vi "RemoteControlForFTJH.vi"() -> ()   [LabVIEW 2020]
uses:
  LMH-PS4/Private/Type Defs/Indicators/Controller.ctl
  LMH-PS4/Private/Type Defs/Indicators/Square.ctl
  LMH-PS4/Private/Type Defs/Indicators/X.ctl
  LMH-PS4/Private/Type Defs/Indicators/Circle.ctl
  LMH-PS4/Private/Type Defs/Indicators/Triangle.ctl
  LMH-PS4/Private/Type Defs/Indicators/L1.ctl
  LMH-PS4/Private/Type Defs/Indicators/R1.ctl
  LMH-PS4/Private/Type Defs/Indicators/Share.ctl
  LMH-PS4/Private/Type Defs/Indicators/Options.ctl
  LMH-PS4/Private/Type Defs/Indicators/PS.ctl
  LMH-PS4/Private/Type Defs/Indicators/Pad_Button.ctl
  LMH-PS4/Private/Type Defs/Indicators/Dpad.ctl
  LMH-PS4/Private/Type Defs/Indicators/Slider.ctl
  <vilib>/Platform/TimedLoop/XDataNode/timing_clust.ctl
  <vilib>/Platform/TimedLoop/XDataNode/nitl_modes.ctl
  <vilib>/Platform/TimedLoop/XDataNode/wakeup.ctl
  <vilib>/CISH Robotics/L4VMX TitanQuad/Motor ID.ctl
  <vilib>/CISH Robotics/L4VMX VMXpi/Type Def/VMX Channel Index.ctl
  servoName.ctl
  <vilib>/CISH Robotics/L4VMX VMXpi/Digital Output/Digital Output.lvclass
  <vilib>/CISH Robotics/L4VMX TitanQuad/TitanQuad.lvclass
  <vilib>/CISH Robotics/L4VMX VMXpi/PWM Generator/PWM Generator.lvclass
  <vilib>/platform/TimedLoop/XDataNode/XDataNode.xnode
  <vilib>/ReMiSYS Technology/RemoteToolkit/Receiver/Receiver.lvclass
  LMH-PS4/LMH-PS4.lvlib
  <vilib>/CISH Robotics/L4VMX VMXpi/Power/Power.lvclass
  <vilib>/Platform/TimedLoop/XDataNode/XDNodeRunTimeDep.lvlib
  <vilib>/CISH Robotics/L4VMX VMXpi/L4VMX.lvlib
  <vilib>/CISH Robotics/L4VMX VMXpi/Utilities/Utilities.lvclass
  <vilib>/CISH Robotics/L4VMX VMXpi/Digital Input/Digital Input.lvclass
panel:
  in  "NormalizeTo":dbl=450.0
  out "Start":bool
  out "Voltage":sgl
  out "Error Out":errorcluster
  in  "Stop":bool
  out "Received?":bool
  out "PS4 Controller":T1={"Square Button"=FALSE, "X Button"=FALSE, "Circle Button"=FALSE, "Triangle Button"=FALSE, "L1"=FALSE, "R1"=FALSE, "Share Button"=FALSE, "Options Button"=FALSE, "PS Button"=FALSE, "Pad Button"=FALSE, "D-Pad"=5, "L2"=0, "R2"=0, "Thumbstick_Left"={[], []}, "Thumbstick_Right"={[], []}} {"R2" scale=-32768.0..32767.0; "L2" scale=-32768.0..32767.0}
  # "ss"
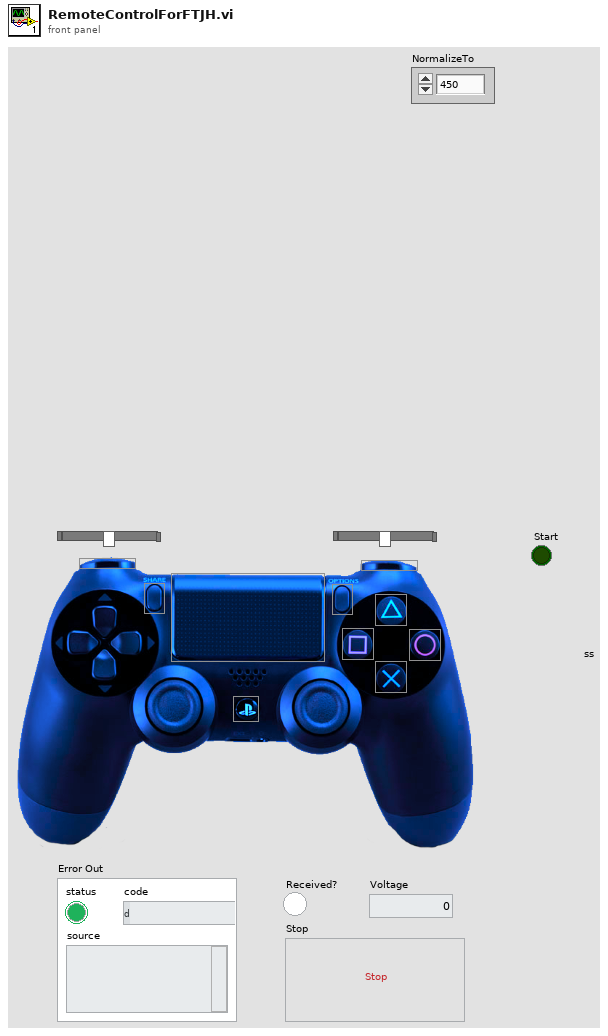
[diagram p1: front panel]
types:
  T1 = typedef "LMH-PS4.lvlib/Controller.ctl" = cluster{"Square Button":T2, "X Button":T3, "Circle Button":T4, "Triangle Button":T5, "L1":T6, "R1":T7, "Share Button":T8, "Options Button":T9, "PS Button":T10, "Pad Button":T11, "D-Pad":T12, "L2":T13, "R2":T13, "Thumbstick_Left":cluster{i32[], i32[]}, "Thumbstick_Right":cluster{i32[], i32[]}}
  T2 = typedef "LMH-PS4.lvlib/Square.ctl" = bool
  T3 = typedef "LMH-PS4.lvlib/X.ctl" = bool
  T4 = typedef "LMH-PS4.lvlib/Circle.ctl" = bool
  T5 = typedef "LMH-PS4.lvlib/Triangle.ctl" = bool
  T6 = typedef "LMH-PS4.lvlib/L1.ctl" = bool
  T7 = typedef "LMH-PS4.lvlib/R1.ctl" = bool
  T8 = typedef "LMH-PS4.lvlib/Share.ctl" = bool
  T9 = typedef "LMH-PS4.lvlib/Options.ctl" = bool
  T10 = typedef "LMH-PS4.lvlib/PS.ctl" = bool
  T11 = typedef "LMH-PS4.lvlib/Pad_Button.ctl" = bool
  T12 = typedef "LMH-PS4.lvlib/Dpad.ctl" = u16
  T13 = typedef "LMH-PS4.lvlib/Slider.ctl" = i32
  T14 = typedef "L4VMX.lvlib/VMX Channel Index.ctl" = enum16{"0", "1", "2", "3", "4", "5", "6", "7", "8", "9", "10", "11", "12", "13", "14", "15", "16", "17", "18", "19", "20", "21", "22", "23", "24", "25", "26", "27", "28", "29", "30", "31", "32", "33"}
  T15 = typedef "TitanQuad.lvlib/TitanQuad.lvclass/Motor ID.ctl" = enum16{"M0", "M1", "M2", "M3"}
  T16 = typedef "XDNodeRunTimeDep.lvlib/timing_clust.ctl" = cluster{"Expected End [f-1]":u64, "Actual End [f-1]":u64, "Finished Late? [f-1]":bool, "Expected End [i-1]":u64, "Actual End [i-1]":u64, "Finished Late? [i-1]":bool, "Expected Start [i]":u64, "Actual Start [i]":u64, "Expected Start [f]":u64, "Actual Start [f]":u64, "Source Name":string, "Structure Name":string, "Period":i64, "Deadline":i64, "Offset":i64, "Start":i64, "Priority":i32, "Timeout":i32, "Mode":T17, "Wakeup Reason":T18, "Error":errorcluster, "Source Type":string, "Secondary Source Type":string, "Global End Time":u64, "Global Start Time":u64, "Frame Duration":u64, "Iteration Duration":u64, "Assigned CPU":i32, "I/O Scan Engine Mode":u32}
  T17 = typedef "XDNodeRunTimeDep.lvlib/nitl_modes.ctl" = enum32{"No Change", "Process missed periods, maintain original phase", "Discard missed periods, maintain original phase", "Process missed periods, ignore original phase", "Discard missed periods, ignore original phase"}
  T18 = typedef "XDNodeRunTimeDep.lvlib/wakeup.ctl" = enum32{"Normal", "Aborted", "Asynchronous wakeup", "Timing source error", "Timed loop error", "Timeout"}
  T19 = typedef "servoName.ctl" = enum16{"Servo1", "Servo2", "Servo3", "Servo4"}
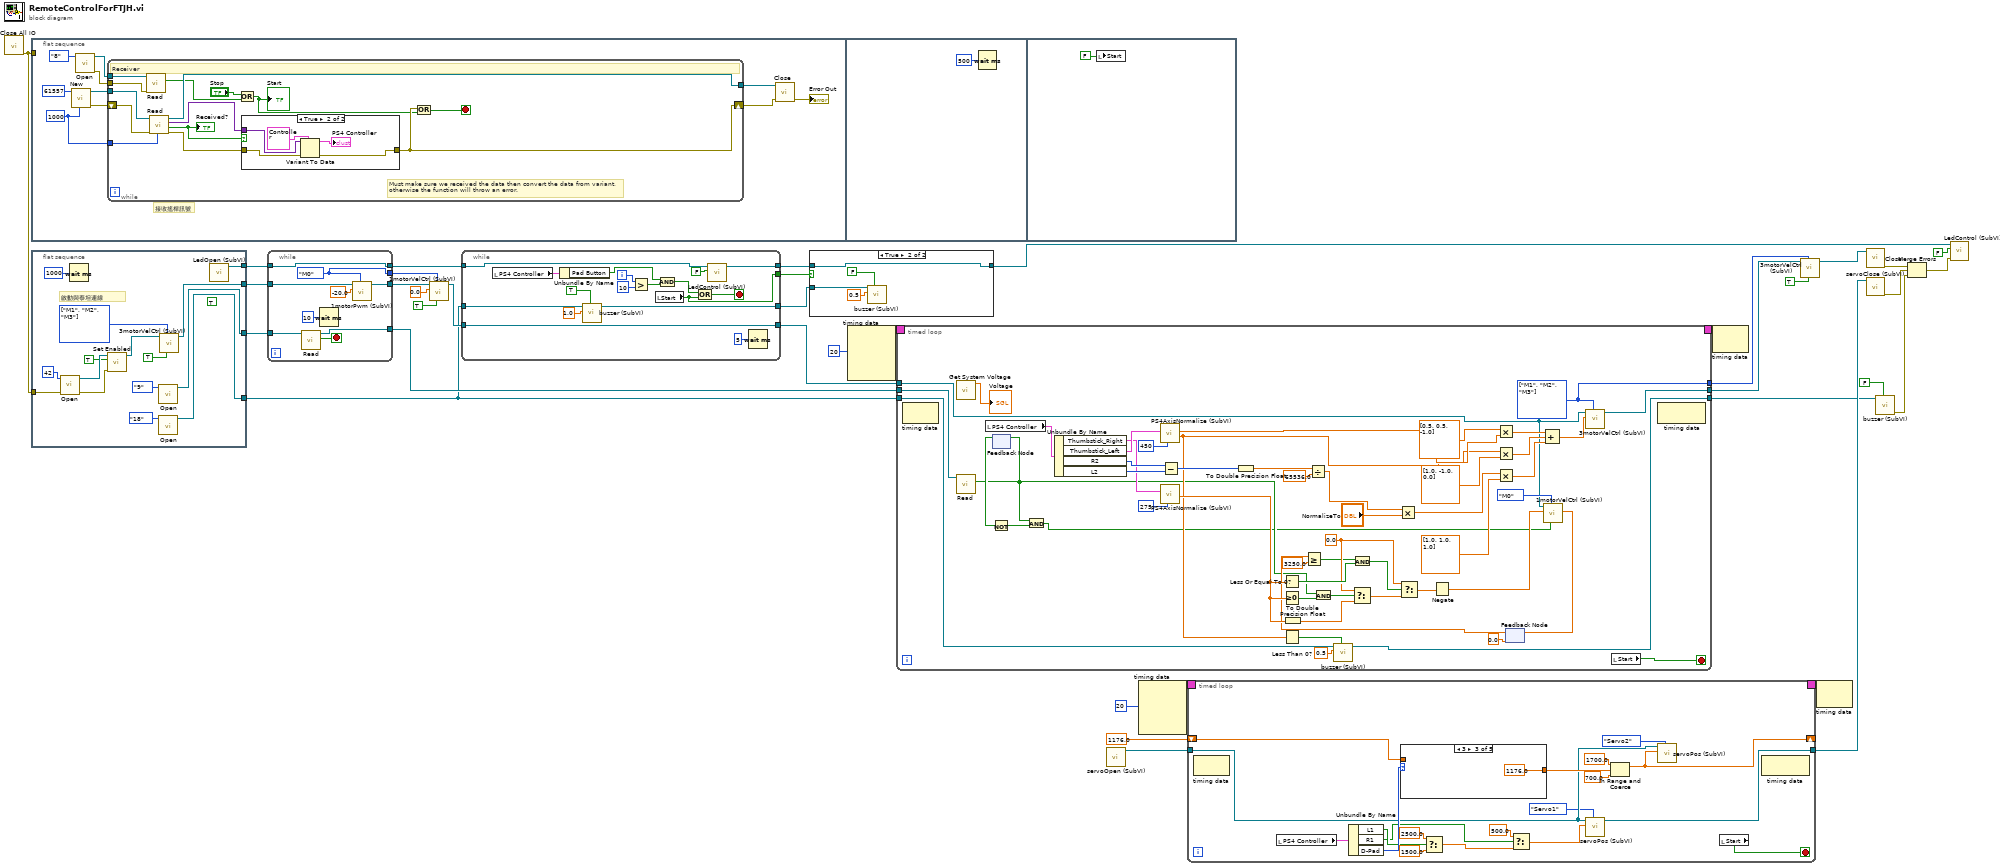
[diagram p0: block diagram]
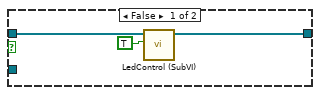
[diagram p2: hidden frame]
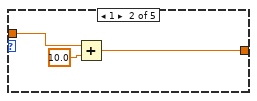
[diagram p4: hidden frame]
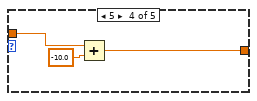
[diagram p5: hidden frame]
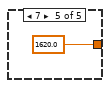
[diagram p6: hidden frame]
diagram:
  n1 = call <vilib>:"Close All IO.vi"() -> ("Error Out"=w1:errorcluster)  [unwired: 11 in]
  n2 = flat-sequence {
    tunnel: w1 -> [_]
    frame #0 {
      w43 = 1000 ("Timeout ms (25000)")
      # "接收搖桿訊號"
      n3 = call <vilib>:"New.vi"("Timeout ms (25000)"=w43, "Port (61557)"=u16 61557) -> ("Error Out"=w47:errorcluster, "Receiver Ref."=w46:refnum<class "Receiver.lvclass">)  [unwired: 8 in]
      n4 = call <vilib>:"Open.vi"("VMX Channel Index"=VMX_Channel_Index."8") -> ("Error Out"=w38:errorcluster, "Digital Input Object"=w39:refnum<class "Digital Input.lvclass">)  [unwired: 9 in]
      n5 = while {
        shift-right: [w54] -> w45
        shift-left: w47 -> [w61]
        tunnel: w46 -> [w60]
        tunnel: [w59] -> w44
        tunnel: w43 -> [w58]
        tunnel: w39 -> [w52]
        tunnel: w38 -> [w51]
        stop <- w57 stop-if-true
        # "Must make sure we received the data then convert the data from variant,\notherwise the function will throw an error."
        # "Receiver"
        n6 = call <vilib>:"Read.vi"("Error In"=w51, "Digital Input Object"=w52) -> ("Value"=w50:bool)  [unwired: 7 in, 2 out]
        n7 = call <vilib>:"Read.vi"("Timeout ms (1000)"=w58, "Error In"=w61, "Receiver Ref."=w60) -> ("Error Out"=w56:errorcluster, "Received?"=w53:bool, "Value"=w55:variant, "Receiver Ref."=w59:refnum<class "Receiver.lvclass">)  [unwired: 5 in]
        "Received?" <- w53
        n8 = Or(x="Stop", y=w50) -> (x .or. y?=w48:bool)
        "Start" <- w48
        n9 = case shown="True" w53 {
          tunnel: w56 -> [w62 w67]
          tunnel: w55 -> [_ w66]
          tunnel: [w62 w65] -> w54
          frame False {
          }
          frame True {
            n10 = Variant To Data(error in=w67, type=T1 {"Square Button"=FALSE, "X Button"=FALSE, "Circle Button"=FALSE, "Triangle Button"=FALSE, "L1"=FALSE, "R1"=FALSE, "Share Button"=FALSE, "Options Button"=FALSE, "PS Button"=FALSE, "Pad Button"=FALSE, "D-Pad"=0, "L2"=-32768, "R2"=-32768, "Thumbstick_Left"={[0, 0], [0, 0]}, "Thumbstick_Right"={[0, 0], [0, 0]}} ("PS4 Controller"), Variant=w66) -> (data=→"PS4 Controller":T1, error out=w65:errorcluster)
          }
        }
        n11 = Or(x=w54, y=w48) -> (x .or. y?=w57:bool)
      }
      n12 = call <vilib>:"Close.vi"("Error In"=w45, "Receiver Ref."=w44) -> ("Error Out"=→"Error Out":errorcluster)  [unwired: 9 in]
    }
    frame #1 {
      n13 = Wait (ms)(milliseconds to wait=u32 500) -> ()  [unwired: 1 out]
    }
    frame #2 {
      n14 = local write "Start"(FALSE ("Stop")) -> ()
    }
  }
  n15 = flat-sequence {
    tunnel: w1 -> [w79]
    tunnel: [w77] -> w10
    tunnel: [w75] -> w12
    tunnel: [w72] -> w3
    tunnel: [w70] -> w2
    frame #0 {
      (unwired) TRUE ("reset Encoder")
      w76 = T15[] [enum."M1", enum."M2", enum."M3"] items=["M0", "M1", "M2", "M3"] ("motorPort [M0, M1, M2]")
      # "啟動與泰坦連線"
      n16 = call <vilib>:"Open.vi"("Error In"=w79, "Titan ID (42)"=u8 42) -> ("Error Out"=w83:errorcluster, "TitanQuad Object"=w84:refnum<class "TitanQuad.lvclass">)  [unwired: 8 in]
      n17 = Wait (ms)(milliseconds to wait=u32 1000) -> ()  [unwired: 1 out]
      n18 = call <vilib>:"Set Enabled.vi"("Error In"=w83, "Enable"=TRUE, "TitanQuad Object"=w84) -> ("TitanQuad Object"=w74:refnum<class "TitanQuad.lvclass">)  [unwired: 7 in, 1 out]
      n19 = call <vilib>:"Open.vi"("VMX Channel Index"=VMX_Channel_Index."9") -> ("Digital Input Object"=w72:refnum<class "Digital Input.lvclass">)  [unwired: 9 in, 1 out]
      n20 = call <vilib>:"Open.vi"("VMX Channel Index"=VMX_Channel_Index."18") -> ("Digital Output Object"=w70:refnum<class "Digital Output.lvclass">)  [unwired: 9 in, 1 out]
      n21 = call "3motorVelCtrl (SubVI).vi"("reset Encoder"=TRUE, "motorPort [M0, M1, M2]"=w76, "TitanQuad in"=w74) -> ("TitanQuad out"=w77:refnum<class "TitanQuad.lvclass">)  [unwired: 6 in, 2 out]
      n22 = call "LedOpen (SubVI).vi"() -> ("LedRef"=w75:refnum<class "Digital Output.lvclass">[])  [unwired: 10 in, 1 out]
    }
  }
  n23 = while {
    tunnel: [w93] -> w13
    tunnel: w12 -> [w93]
    tunnel: [w90] -> w8
    tunnel: w10 -> [w92]
    tunnel: [w89] -> w9
    tunnel: w3 -> [w88]
    tunnel: [w87] -> w4
    stop <- w86 stop-if-true
    w89 = Motor_ID."M0" ("Motor ID")
    n24 = call <vilib>:"Read.vi"("Digital Input Object"=w88) -> ("Value"=w86:bool, "Digital Input Object"=w87:refnum<class "Digital Input.lvclass">)  [unwired: 8 in, 1 out]
    n25 = Wait (ms)(milliseconds to wait=u32 10) -> ()  [unwired: 1 out]
    n26 = call "1motorPwm (SubVI).vi"("Motor ID"=w89, "motorPwmSpeed"=-20.0, "TitanQuad in"=w92) -> ("TitanQuad out"=w90:refnum<class "TitanQuad.lvclass">)  [unwired: 6 in, 2 out]
  }
  n27 = call "1motorVelCtrl (SubVI).vi"("reset Encoder"=TRUE, "Motor ID"=w9, "motorSpeed (deg/s)"=0.0, "TitanQuad in"=w8) -> ("TitanQuad out"=w7:refnum<class "TitanQuad.lvclass">)  [unwired: 3 in, 4 out]
  n28 = while {
    tunnel: [w102] -> w30
    tunnel: w13 -> [w101]
    tunnel: [w99] -> w23
    tunnel: w2 -> [w98]
    tunnel: [w96] -> w14
    tunnel: [w94] -> w11
    tunnel: w7 -> [w94]
    i -> [w107]
    stop <- w103 stop-if-true
    n29 = local read "PS4 Controller"() -> (w110:T1)
    n30 = Unbundle By Name(w110) -> ("Pad Button"=w108:T11)
    n31 = call "buzzer (SubVI).vi"("BuzzerOn"=TRUE, "Time Target (s)"=1.0, "Digital Output in"=w98) -> ("Digital Output out"=w96:refnum<class "Digital Output.lvclass">)  [unwired: 7 in, 1 out]
    n32 = Greater?(x=w107, y=10) -> (0:w105:bool)
    n33 = local read "Start"() -> (w102:bool)
    n34 = And(x=w108, y=w105) -> (x .and. y?=w104:T11)
    n35 = Or(x=w104, y=w102) -> (x .or. y?=w103:T11)
    n36 = call "LedControl (SubVI).vi"("Red/Green [T/F]"=FALSE, "LedRef"=w101) -> ("LedRef"=w99:refnum<class "Digital Output.lvclass">[])  [unwired: 8 in, 1 out]
    n37 = Wait (ms)(milliseconds to wait=u32 5) -> ()  [unwired: 1 out]
  }
  n38 = case shown="True" w30 {
    tunnel: w23 -> [w112 w117]
    tunnel: [w111 w117] -> w20
    tunnel: w14 -> [_ w115]
    frame False {
      n39 = call "LedControl (SubVI).vi"("Red/Green [T/F]"=TRUE, "LedRef"=w112) -> ("LedRef"=w111:refnum<class "Digital Output.lvclass">[])  [unwired: 8 in, 1 out]
    }
    frame True {
      n40 = call "buzzer (SubVI).vi"("BuzzerOn"=FALSE, "Time Target (s)"=0.5, "Digital Output in"=w115) -> ()  [unwired: 7 in, 2 out]
    }
  }
  n41 = node-c288(i64 20 ("Period")) -> (w37:T16)  [unwired: 3 in]
  n42 = timed-loop {
    timing: w37 -> [_]
    timing-out: [_] -> w36
    tunnel: w4 -> [w158]
    tunnel: [w148] -> w29
    tunnel: [w147] -> w26
    tunnel: w2 -> [w130]
    tunnel: [w127] -> w17
    tunnel: w11 -> [w125]
    stop <- w169 stop-if-true
    w147 = T15[] [enum."M1", enum."M2", enum."M3"] items=["M0", "M1", "M2", "M3"] ("motorPort [M0, M1, M2]")
    w152 = 0.0 ("t")
    n43 = node-c288() -> ()  [unwired: 1 in, 1 out]
    n44 = call <vilib>:"Get System Voltage.vi"() -> ("Voltage"=→"Voltage":sgl)  [unwired: 10 in, 1 out]
    n45 = call <vilib>:"Read.vi"("Digital Input Object"=w158) -> ("Value"=w122:bool)  [unwired: 8 in, 2 out]
    n46 = local read "PS4 Controller"() -> (w167:T1)
    n47 = feedback-in #1(w122) -> ()
    n48 = feedback #1() -> (w123:bool)  [unwired: 1 in]
    n49 = Not(x=w123) -> (.not. x?=w124:bool)
    n50 = And(x=w122, y=w124) -> (x .and. y?=w121:bool)
    n51 = Unbundle By Name(w167) -> ("Thumbstick_Right"=w140:cluster{i32[], i32[]}, "Thumbstick_Left"=w143:cluster{i32[], i32[]}, "R2"=w166:T13, "L2"=w165:T13)
    n52 = call "PS4AxisNormalize (SubVI).vi"("NormalizeTo"=450, "PS4 Thumbstick"=w143) -> ("Y"=w129:dbl, "X"=w142:dbl)  [unwired: 8 in]
    n53 = call "PS4AxisNormalize (SubVI).vi"("NormalizeTo"=275, "PS4 Thumbstick"=w140) -> ("Y"=w138:dbl)  [unwired: 8 in, 1 out]
    n54 = Subtract(x=w166, y=w165) -> (x-y=w131:T13)
    n55 = To Double Precision Float(number=w131) -> (double precision float=w133:dbl)
    n56 = Less Or Equal To 0?(x=w138) -> (x <= 0?=w154:bool)
    n57 = Greater Or Equal To 0?(x=w138) -> (x >= 0?=w157:bool)
    n58 = Less Than 0?(x=w129) -> (x < 0?=w128:bool)
    n59 = To Double Precision Float(number=w138) -> (double precision float=w137:dbl)
    n60 = Divide(x=w133, y=65536.0) -> (x/y=w120:dbl)
    n61 = And(x=w122, y=w157) -> (x .and. y?=w156:bool)
    n62 = call "buzzer (SubVI).vi"("BuzzerOn"=w128, "Time Target (s)"=0.5, "Digital Output in"=w130) -> ("Digital Output out"=w127:refnum<class "Digital Output.lvclass">)  [unwired: 7 in, 1 out]
    n63 = Select(t=w152, s=w156, f=w137) -> (s? t:f=w155:dbl)
    n64 = Multiply(x=w120, y="NormalizeTo") -> (x*y=w118:dbl)
    n65 = Multiply(x=dbl[] [0.5, 0.5, -1.0], y=w142) -> (x*y=w161:dbl[])
    n66 = Multiply(x=w129, y=dbl[] [1.0, -1.0, 0.0]) -> (x*y=w160:dbl[])
    n67 = Multiply(x=w118, y=dbl[] [1.0, 1.0, 1.0]) -> (x*y=w164:dbl[])
    n68 = feedback #2(0.0 ("Enc (deg)")) -> (w135:dbl)
    n69 = Greater Or Equal?(x=w135, y=3250.0) -> (x >= y?=w150:bool)
    n70 = And(x=w150, y=w154) -> (x .and. y?=w153:bool)
    n71 = Select(t=w152, s=w153, f=w155) -> (s? t:f=w145:dbl)
    n72 = Negate(x=w145) -> (-x=w144:dbl)
    n73 = call "1motorVelCtrl (SubVI).vi"("reset Encoder"=w121, "Motor ID"=Motor_ID."M0", "motorSpeed (deg/s)"=w144, "TitanQuad in"=w125) -> ("Enc (deg)"=w136:dbl)  [unwired: 3 in, 4 out]
    n74 = feedback-in #2(w136) -> ()
    n75 = Compound Arithmetic op=ADD(w161, w160, w164) -> (w149:dbl[])
    n76 = call "3motorVelCtrl (SubVI).vi"("motorPort [M0, M1, M2]"=w147, "motorSpeed [M0, M1, M2] (deg/s)"=w149, "TitanQuad in"=w125) -> ("TitanQuad out"=w148:refnum<class "TitanQuad.lvclass">)  [unwired: 6 in, 2 out]
    n77 = local read "Start"() -> (w169:bool)
    n78 = node-c288() -> ()  [unwired: 1 in, 1 out]
  }
  n79 = call "servoOpen (SubVI).vi"() -> ("ServosRef"=w25:refnum<class "PWM Generator.lvclass">[])  [unwired: 10 in, 1 out]
  n80 = node-c288(i64 20 ("Period")) -> (w34:T16)  [unwired: 3 in]
  n81 = timed-loop {
    timing: w34 -> [_]
    timing-out: [_] -> w33
    shift-right: [w172] -> _
    shift-left: 1176.0 ("y") -> [w187]
    tunnel: w25 -> [w178]
    tunnel: [w177] -> w24
    stop <- w190 stop-if-true
    n82 = node-c288() -> ()  [unwired: 1 in, 1 out]
    n83 = local read "PS4 Controller"() -> (w189:T1)
    n84 = Unbundle By Name(w189) -> ("L1"=w183:T6, "R1"=w175:T7, "D-Pad"=w188:T12)
    n85 = case shown="3" w188 {
      tunnel: w187 -> [w191 w194 _ w198 _]
      tunnel: [w191 w192 1176.0 ("y") w196 1620.0 ("y")] -> w185
      frame 0, Default {
      }
      frame 1 {
        n86 = Add(x=w194, y=10.0) -> (x+y=w192:dbl)
      }
      frame 3 {
      }
      frame 5 {
        n87 = Add(x=w198, y=-10.0) -> (x+y=w196:dbl)
      }
      frame 7 {
      }
    }
    n88 = Select(t=2500.0, s=w183, f=1500.0 ("lower limit")) -> (s? t:f=w181:dbl)
    n89 = Select(t=500.0, s=w175, f=w181) -> (s? t:f=w174:dbl)
    n90 = call "servoPos (SubVI).vi"("Servos"=servoName."Servo1", "ServoPosition (us)"=w174, "ServosRef in"=w178) -> ("ServosRef out"=w177:refnum<class "PWM Generator.lvclass">[])  [unwired: 7 in, 1 out]
    n91 = In Range and Coerce(upper limit=1700.0, x=w185, lower limit=700.0) -> (coerced(x)=w172:dbl)  [unwired: 1 out]
    n92 = call "servoPos (SubVI).vi"("Servos"=servoName."Servo2", "ServoPosition (us)"=w172, "ServosRef in"=w178) -> ()  [unwired: 7 in, 2 out]
    n93 = local read "Start"() -> (w190:bool)
    n94 = node-c288() -> ()  [unwired: 1 in, 1 out]
  }
  n95 = node-c288(w36) -> ()  [unwired: 1 out]
  n96 = call "3motorVelCtrl (SubVI).vi"("reset Encoder"=TRUE, "motorPort [M0, M1, M2]"=w26, "TitanQuad in"=w29) -> ("TitanQuad out"=w28:refnum<class "TitanQuad.lvclass">)  [unwired: 6 in, 2 out]
  n97 = node-c288(w33) -> ()  [unwired: 1 out]
  n98 = call <vilib>:"Close.vi"("TitanQuad Object"=w28) -> ("Error Out"=w22:errorcluster)  [unwired: 10 in]
  n99 = call "servoClose (SubVI).vi"("ServosRef"=w24) -> ("error out"=w21:errorcluster)  [unwired: 10 in]
  n100 = call "buzzer (SubVI).vi"("BuzzerOn"=FALSE, "Digital Output in"=w17) -> ("Error Out"=w16:errorcluster)  [unwired: 8 in, 1 out]
  n101 = Merge Errors(w22, w21, w16) -> (w19:errorcluster)
  n102 = call "LedControl (SubVI).vi"("error in (no error)"=w19, "Red/Green [T/F]"=FALSE, "LedRef"=w20) -> ()  [unwired: 7 in, 2 out]
